vi "Read Key Ref.vi"(6 "Key Name":string, 7 "Section":string, 8 "error in (no error)":errorcluster, 10 "Section Element":variant, 11 "Refnum in":T1) -> (0 "error out":errorcluster, 1 "found?":bool, 2 "Variant Element Data":variant, 3 "Refnum out":T1, 4 "Key Name out":string)   [LabVIEW 2024, in "Generic Config Handling.lvlib"]
doc: "This vi reads a variant to a config file.\n\nIt only accepts very basic datatypes. \n\nIt will accept 1D and 2D arrays.\n\nIf key name is not wired, then it will use the name of the section element.\n\nSection Element in provides the type information and the default value."
uses:
  Generic Config Handling.lvlib
  <vilib>/Utility/config.llb/Config Data RefNum.ctl
  <vilib>/Utility/config.llb/Read Key (I32).vi
  <vilib>/Utility/config.llb/Read Key (U32).vi
  <vilib>/Utility/config.llb/Read Key (Double).vi
  <vilib>/Utility/config.llb/Read Key (Boolean).vi
  <vilib>/Utility/config.llb/Read Key (String).vi
  <vilib>/Utility/config.llb/Read Key (Path).vi
  <vilib>/Utility/VariantDataType/VariantType.lvlib
  <vilib>/Utility/config.llb/NI_LVConfig.lvlib
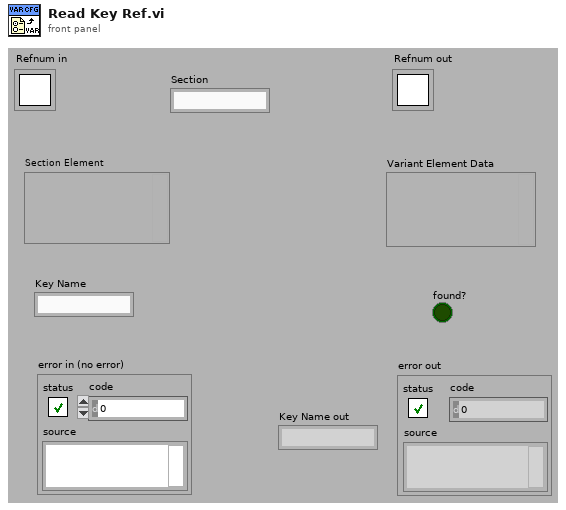
[diagram p1: front panel]
types:
  T1 = typedef "NI_LVConfig.lvlib/Config Data RefNum.ctl" = refnum<k1>
  T2 = typedef "VariantType.lvlib/Type.ctl" = enum8{"Invalid Type", "Void", "I8", "I16", "I32", "I64", "U8", "U16", "U32", "U64", "Single Float", "Double Float", "Extended Float", "Single Complex", "Double Complex", "Extended Complex", "Enum U8", "Enum U16", "Enum U32", "Enum U64", "Single Float With Unit", "Double Float With Unit", "Extended Float With Unit", "Single Complex with Unit", "Double Complex with Unit", "Extended Complex with Unit", "Boolean", "String", "Path", "Picture", "Tag", "Array", "Cluster", "Variant", "LV Variant", "Waveform", "Timestamp", "Digital Waveform", "Digital Data", "ExpressData", "Refnum", "External Data", "VI", "Poly VI", "LabVIEW Class Instance", "Fixed Point"}
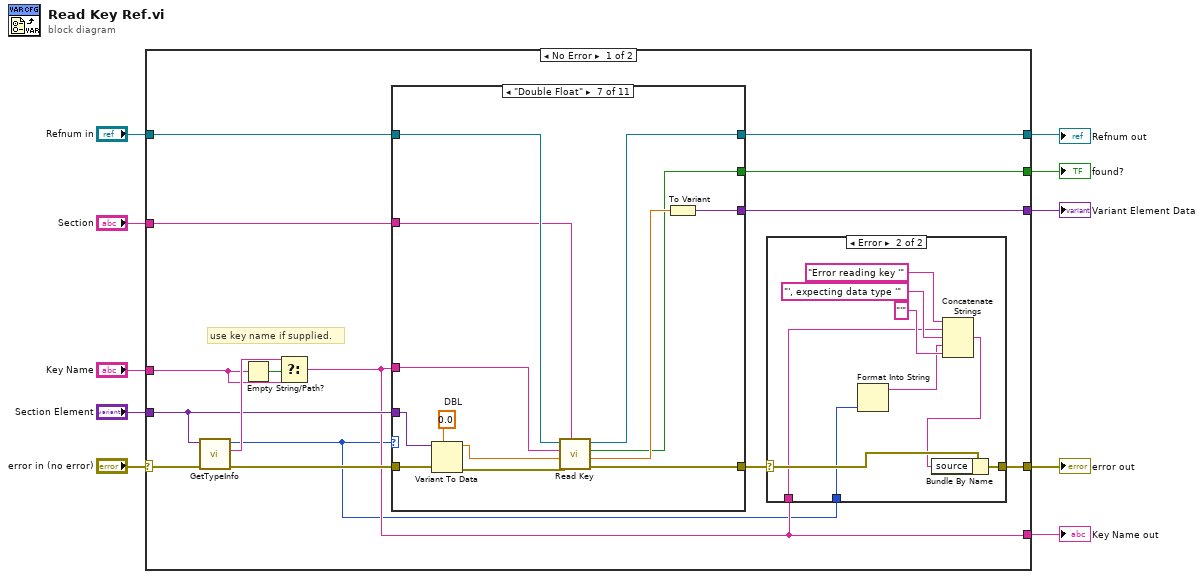
[diagram p0: block diagram]
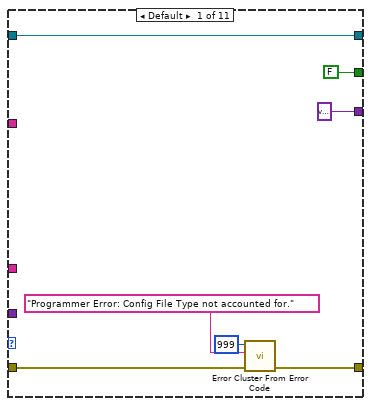
[diagram p3: hidden frame]
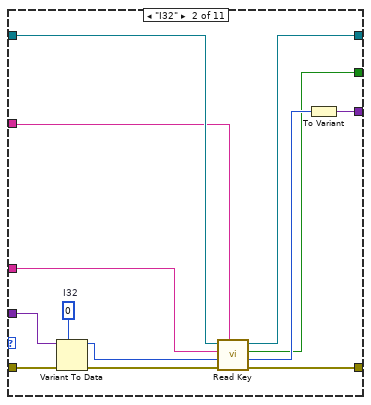
[diagram p4: hidden frame]
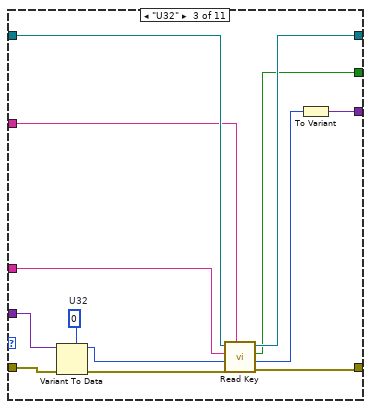
[diagram p5: hidden frame]
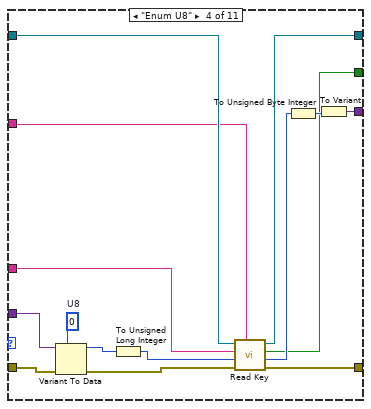
[diagram p6: hidden frame]
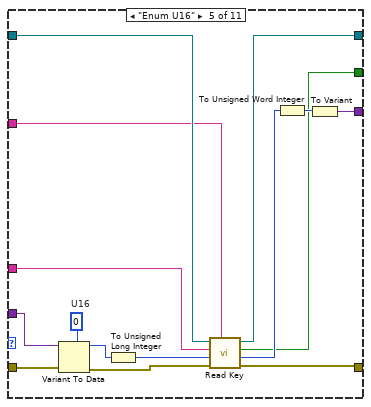
[diagram p7: hidden frame]
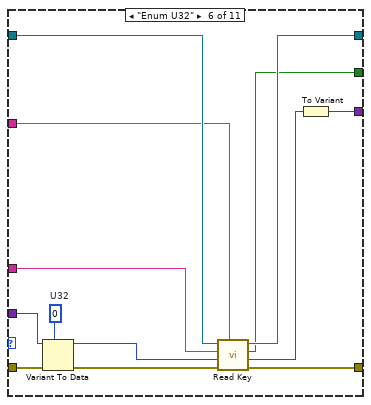
[diagram p8: hidden frame]
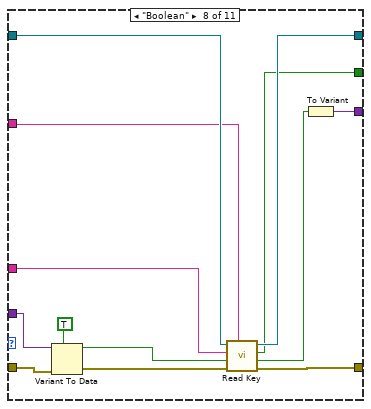
[diagram p9: hidden frame]
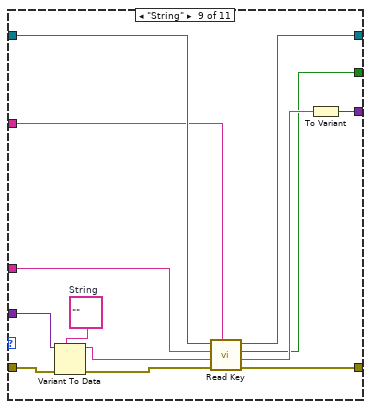
[diagram p10: hidden frame]
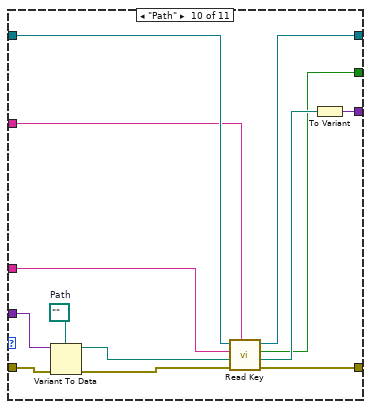
[diagram p11: hidden frame]
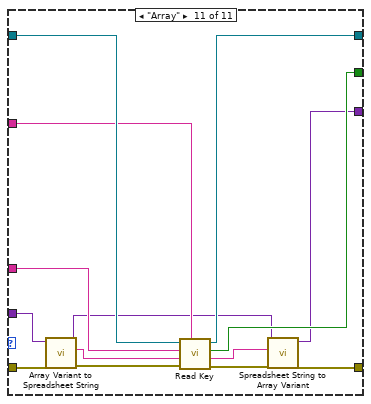
[diagram p12: hidden frame]
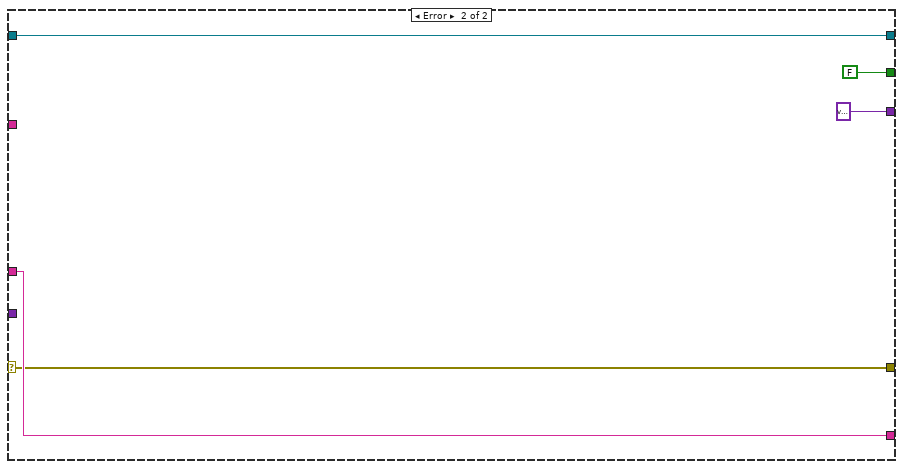
[diagram p13: hidden frame]
diagram:
  n1 = case shown="No Error" "error in (no error)" {
    selector: "error in (no error)" -> [w15 w180]
    tunnel: "Key Name" -> [w23 w181]
    tunnel: [w13 w180] -> w9
    tunnel: "Refnum in" -> [w22 w182]
    tunnel: [w21 w182] -> w7
    tunnel: [w20 variant ("Variant")] -> w6
    tunnel: [w19 FALSE ("found?")] -> w5
    tunnel: "Section Element" -> [w18 _]
    tunnel: "Section" -> [w17 _]
    tunnel: [w12 w181] -> w2
    frame No Error {
      # "use key name if supplied."
      n2 = call <vilib>:"GetTypeInfo.vi"("error in (no error)"=w15, "Variant"=w18) -> ("error out"=w16:errorcluster, "Name"=w24:string, "Type Enum"=w11:T2)  [unwired: 5 in, 2 out]
      n3 = Empty String/Path?(string/path=w23) -> (empty?=w25:bool)
      n4 = Select(t=w24, s=w25, f=w23) -> (s? t:f=w12:string)
      n5 = case shown="\"Double Float\"" w11 {
        tunnel: w16 -> [w40 w44 w56 w72 w86 w101 w113 w126 w139 w152 w176]
        tunnel: w12 -> [_ w51 w64 w79 w94 w107 w120 w133 w143 w159 w174]
        tunnel: [w39 w53 w66 w81 w96 w109 w122 w135 w148 w161 w168] -> w14
        tunnel: w22 -> [w38 w55 w68 w83 w98 w111 w124 w137 w150 w163 w175]
        tunnel: [w38 w54 w67 w82 w97 w110 w123 w136 w149 w162 w171] -> w21
        tunnel: w17 -> [_ w52 w65 w80 w95 w108 w121 w134 w147 w160 w172]
        tunnel: [variant ("Variant") w49 w62 w77 w92 w106 w118 w131 w145 w157 w167] -> w20
        tunnel: [FALSE ("found?") w48 w61 w75 w90 w105 w117 w130 w144 w156 w170] -> w19
        tunnel: w18 -> [_ w47 w59 w73 w87 w103 w115 w128 w141 w154 w177]
        frame Default {
          n6 = call <vilib>:"Error Cluster From Error Code.vi"("error in (no error)"=w40, "error message (\"\")"="Programmer Error: Config File Type not accounted for." ("error message (\"\")"), "error code (0)"=999) -> ("error out"=w39:errorcluster)  [unwired: 6 in]
        }
        frame "I32" {
          w46 = 0  # I32
          n7 = Variant To Data(error in=w44, type=w46, Variant=w47) -> (data=w45:i32, error out=w43:errorcluster)
          n8 = call-poly <vilib>:"Read Key.vi"("section"=w52, "error in (no error)"=w43, "default value"=w45, "key"=w51, "refnum"=w55) -> ("error out"=w53:errorcluster, "value"=w50:i32, "found?"=w48:bool, "refnum out"=w54:T1)  [unwired: 3 in]
          n9 = To Variant(anything=w50) -> (Variant=w49:variant)
        }
        frame "U32" {
          w60 = u32 0  # U32
          n10 = Variant To Data(error in=w56, type=w60, Variant=w59) -> (data=w58:u32, error out=w57:errorcluster)
          n11 = call-poly <vilib>:"Read Key.vi"("section"=w65, "error in (no error)"=w57, "default value"=w58, "key"=w64, "refnum"=w68) -> ("error out"=w66:errorcluster, "value"=w63:u32, "found?"=w61:bool, "refnum out"=w67:T1)  [unwired: 3 in]
          n12 = To Variant(anything=w63) -> (Variant=w62:variant)
        }
        frame "Enum U8" {
          w74 = u8 0  # U8
          n13 = Variant To Data(error in=w72, type=w74, Variant=w73) -> (data=w70:u8, error out=w71:errorcluster)
          n14 = To Unsigned Long Integer(number=w70) -> (unsigned 32bit integer=w69:u32)
          n15 = call-poly <vilib>:"Read Key.vi"("section"=w80, "error in (no error)"=w71, "default value"=w69, "key"=w79, "refnum"=w83) -> ("error out"=w81:errorcluster, "value"=w78:u32, "found?"=w75:bool, "refnum out"=w82:T1)  [unwired: 3 in]
          n16 = To Unsigned Byte Integer(number=w78) -> (unsigned 8bit integer=w76:u8)
          n17 = To Variant(anything=w76) -> (Variant=w77:variant)
        }
        frame "Enum U16" {
          w89 = u16 0  # U16
          n18 = Variant To Data(error in=w86, type=w89, Variant=w87) -> (data=w88:u16, error out=w85:errorcluster)
          n19 = To Unsigned Long Integer(number=w88) -> (unsigned 32bit integer=w84:u32)
          n20 = call-poly <vilib>:"Read Key.vi"("section"=w95, "error in (no error)"=w85, "default value"=w84, "key"=w94, "refnum"=w98) -> ("error out"=w96:errorcluster, "value"=w93:u32, "found?"=w90:bool, "refnum out"=w97:T1)  [unwired: 3 in]
          n21 = To Unsigned Word Integer(number=w93) -> (unsigned 16bit integer=w91:u16)
          n22 = To Variant(anything=w91) -> (Variant=w92:variant)
        }
        frame "Enum U32" {
          w104 = u32 0  # U32
          n23 = Variant To Data(error in=w101, type=w104, Variant=w103) -> (data=w102:u32, error out=w100:errorcluster)
          n24 = call-poly <vilib>:"Read Key.vi"("section"=w108, "error in (no error)"=w100, "default value"=w102, "key"=w107, "refnum"=w111) -> ("error out"=w109:errorcluster, "value"=w99:u32, "found?"=w105:bool, "refnum out"=w110:T1)  [unwired: 3 in]
          n25 = To Variant(anything=w99) -> (Variant=w106:variant)
        }
        frame "Double Float" {
          w116 = 0.0  # DBL
          n26 = Variant To Data(error in=w113, type=w116, Variant=w115) -> (data=w114:dbl, error out=w112:errorcluster)
          n27 = call-poly <vilib>:"Read Key.vi"("section"=w121, "error in (no error)"=w112, "default value"=w114, "key"=w120, "refnum"=w124) -> ("error out"=w122:errorcluster, "value"=w119:dbl, "found?"=w117:bool, "refnum out"=w123:T1)  [unwired: 3 in]
          n28 = To Variant(anything=w119) -> (Variant=w118:variant)
        }
        frame "Boolean" {
          n29 = Variant To Data(error in=w126, type=TRUE, Variant=w128) -> (data=w127:bool, error out=w125:errorcluster)
          n30 = call-poly <vilib>:"Read Key.vi"("section"=w134, "error in (no error)"=w125, "default value"=w127, "key"=w133, "refnum"=w137) -> ("error out"=w135:errorcluster, "value"=w132:bool, "found?"=w130:bool, "refnum out"=w136:T1)  [unwired: 3 in]
          n31 = To Variant(anything=w132) -> (Variant=w131:variant)
        }
        frame "String" {
          w142 = ""  # String
          n32 = Variant To Data(error in=w139, type=w142, Variant=w141) -> (data=w140:string, error out=w138:errorcluster)
          n33 = call-poly <vilib>:"Read Key.vi"("section"=w147, "error in (no error)"=w138, "default value"=w140, "key"=w143, "refnum"=w150) -> ("error out"=w148:errorcluster, "value"=w146:string, "found?"=w144:bool, "refnum out"=w149:T1)  [unwired: 3 in]
          n34 = To Variant(anything=w146) -> (Variant=w145:variant)
        }
        frame "Path" {
          w155 = path ""  # Path
          n35 = Variant To Data(error in=w152, type=w155, Variant=w154) -> (data=w153:path, error out=w151:errorcluster)
          n36 = call-poly <vilib>:"Read Key.vi"("section"=w160, "error in (no error)"=w151, "default value"=w153, "key"=w159, "refnum"=w163) -> ("error out"=w161:errorcluster, "value"=w158:path, "found?"=w156:bool, "refnum out"=w162:T1)  [unwired: 3 in]
          n37 = To Variant(anything=w158) -> (Variant=w157:variant)
        }
        frame "Array" {
          n38 = call "Array Variant to Spreadsheet String.vi"("error in (no error)"=w176, "Array Variant"=w177) -> ("error out"=w173:errorcluster, "spreadsheet string"=w166:string, "Array Variant  out (dup)"=w165:variant)  [unwired: 7 in]
          n39 = call-poly <vilib>:"Read Key.vi"("section"=w172, "error in (no error)"=w173, "default value"=w166, "key"=w174, "refnum"=w175) -> ("error out"=w169:errorcluster, "value"=w164:string, "found?"=w170:bool, "refnum out"=w171:T1)  [unwired: 3 in]
          n40 = call "Spreadsheet String to Array Variant.vi"("error in (no error)"=w169, "spreadsheet string in"=w164, "Array Variant in (type)"=w165) -> ("error out"=w168:errorcluster, "Array Variant out"=w167:variant)  [unwired: 7 in]
        }
      }
      n41 = case shown="Error" w14 {
        selector: w14 -> [w26 w31]
        tunnel: [w26 w32] -> w13
        tunnel: w12 -> [_ w30]
        tunnel: w11 -> [_ w29]
        frame No Error {
        }
        frame Error {
          n42 = Format Into String(w29) -> (resulting string=w28:string)  [unwired: 3 in, 1 out]
          n43 = Concatenate Strings("Error reading key '" ("string"), w30, "', expecting data type '" ("string"), w28, "'" ("string")) -> (w27:string)
          n44 = Bundle By Name(cluster=w31, "source"=w27) -> (w32:errorcluster)
        }
      }
    }
    frame Error {
    }
  }
  "Refnum out" <- w7
  "error out" <- w9
  "Variant Element Data" <- w6
  "found?" <- w5
  "Key Name out" <- w2
